vi "arrayTypesExample.vi"() -> ()   [LabVIEW 2014]
panel:
  out "Floating Point Array":dbl[][][][][](array[numeric])
  out "String Array":string[][][][][](array[string])
  out "Integer Array":i32[][][][][](array[numeric])
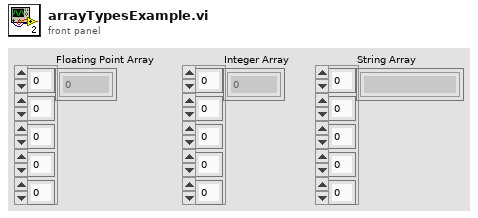
[diagram p1: front panel]
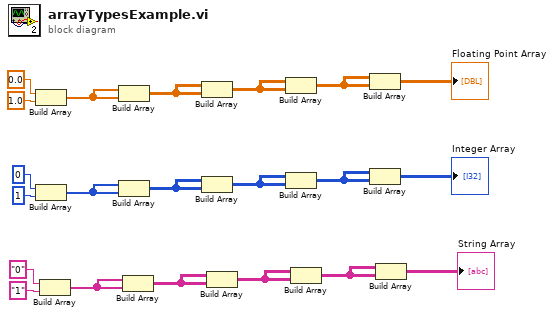
[diagram p0: block diagram]
diagram:
  n1 = Build Array(0.0 ("element"), 1.0 ("element")) -> (w19:dbl[])
  n2 = Build Array(0 ("element"), 1 ("element")) -> (w13:i32[])
  n3 = Build Array("0", "1") -> (w9:string[])
  n4 = Build Array(w19, w19) -> (w18:dbl[][])
  n5 = Build Array(w13, w13) -> (w12:i32[][])
  n6 = Build Array(w9, w9) -> (w8:string[][])
  n7 = Build Array(w18, w18) -> (w17:dbl[][][])
  n8 = Build Array(w12, w12) -> (w11:i32[][][])
  n9 = Build Array(w8, w8) -> (w7:string[][][])
  n10 = Build Array(w17, w17) -> (w16:dbl[][][][])
  n11 = Build Array(w11, w11) -> (w10:i32[][][][])
  n12 = Build Array(w7, w7) -> (w6:string[][][][])
  n13 = Build Array(w16, w16) -> (→"Floating Point Array":dbl[][][][][])
  n14 = Build Array(w10, w10) -> (→"Integer Array":i32[][][][][])
  n15 = Build Array(w6, w6) -> (→"String Array":string[][][][][])
